vi "Convert JSON Time to Timestamp.vi"(11 "JSON Citadel Time string":string) -> (3 "time stamp":timestamp)   [LabVIEW 2019]
uses:
  <vilib>/Utility/miscctls.llb/LVDateTimeRec.ctl
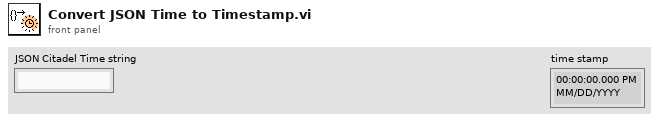
[diagram p1: front panel]
types:
  T1 = typedef "LVDateTimeRec.ctl" = cluster{"fractional second":dbl, "second":i32, "minute":i32, "hour":i32, "day of month":i32, "month":i32, "year":i32, "day of week":i32, "day of year":i32, "DST":i32}
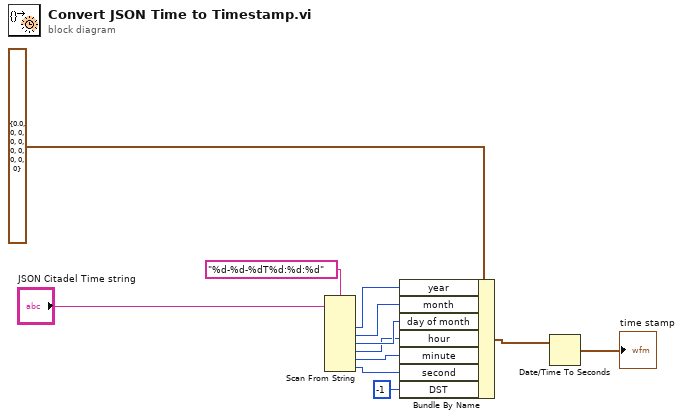
[diagram p0: block diagram]
diagram:
  n1 = Scan From String(format string="%d-%d-%dT%d:%d:%d", input string="JSON Citadel Time string") -> (output 1=w11:i32, output 2=w10:i32, output 3=w9:i32, output 4=w8:i32, output 5=w7:i32, output 6=w6:i32)  [unwired: 8 in, 3 out]
  n2 = Bundle By Name(cluster=T1 {"fractional second"=0.0, "second"=0, "minute"=0, "hour"=0, "day of month"=0, "month"=0, "year"=0, "day of week"=0, "day of year"=0, "DST"=0} ("date time rec"), "year"=w11, "month"=w10, "day of month"=w9, "hour"=w8, "minute"=w7, "second"=w6, "DST"=-1) -> (w3:T1)
  n3 = Date/Time To Seconds(2:w3) -> (0:→"time stamp":timestamp)  [unwired: 1 in]
